vi "Teleop.vi"(10 "Match Info":T1={"Autonomous Elapsed Seconds"=0.0, "TeleOp Elapsed Seconds"=0.0, "Disabled Elapsed Seconds"=0.0, "Visited Autonomous"=FALSE, "Visited TeleOp"=FALSE, "Visited Disabled"=FALSE, "Autonomous Settings"={"Autonomous Style"=enum."Independent", "VI Refnum"=refnum}}, 11 "Call Context":T2) -> ()   [LabVIEW 2017]
doc: "This VI is called for each TeleOp packet received from the DS where the robot is not disabled. It is often used to read from the joysticks and update I/O or to update setpoints for timed control loops. It should complete and return within 20 milliseconds or it may miss DS packets."
uses:
  <vilib>/Rock Robotics/WPI/DriverStation/WPI_DriverStationDerivedRobotMode.ctl
  <vilib>/Rock Robotics/WPI/DriverStation/WPI_DriverStationMatch Info.ctl
  <vilib>/Rock Robotics/WPI/Solenoid/WPI_SolenoidValue.ctl
  <vilib>/Rock Robotics/WPI/Utilities/WPI_GetSetVariantRefNum.vi
  <vilib>/Rock Robotics/Network Tables/NT Write Boolean Array.vi
  <vilib>/Rock Robotics/Network Tables/NT Write Numeric Array.vi
  <vilib>/Rock Robotics/Network Tables/NT Read Boolean.vi
  <vilib>/Rock Robotics/Network Tables/NT Read Number.vi
  <vilib>/Rock Robotics/Network Tables/NT Write Number.vi
  <vilib>/Rock Robotics/WPI/Solenoid/WPI_SolenoidSetEnum.vi
panel:
  out "Sample Slider 0":dbl(slide) scale=0.0..5.0
  out "Sample Boolean 1":bool
  out "Sample Boolean 0":bool
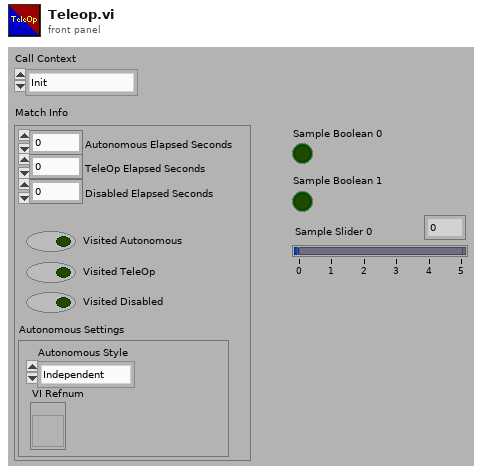
[diagram p1: front panel]
types:
  T1 = typedef "WPI_DriverStationMatch Info.ctl" = cluster{"Autonomous Elapsed Seconds":dbl, "TeleOp Elapsed Seconds":dbl, "Disabled Elapsed Seconds":dbl, "Visited Autonomous":bool, "Visited TeleOp":bool, "Visited Disabled":bool, "Autonomous Settings":cluster{"Autonomous Style":enum16{"Iterative", "Independent"}, "VI Refnum":refnum<vi>}}
  T2 = typedef "WPI_DriverStationDerivedRobotMode.ctl" = enum16{"Init", "Execute", "Stop"}
  T3 = typedef "WPI_SolenoidValue.ctl" = enum16{"Off", "On", "Forward", "Reverse"}
  T4 = typedef "WPI_JoystickDevRef.ctl" = cluster{"Device":T5}
  T5 = typedef "WPI_JoystickDeviceEnum.ctl" = enum16{"USB 0", "USB 1", "USB 2", "USB 3", "USB 4", "USB 5"}
  T6 = cluster{"Axes[0]":dbl, "Axes[1]":dbl, "Axes[2]":dbl, "Axes[3]":dbl, "Axes[4]":dbl, "Axes[5]":dbl, "Axes[6]":dbl, "Axes[7]":dbl, "Axes[8]":dbl}
  T7 = cluster{"Buttons[0]":bool, "Buttons[1]":bool, "Buttons[2]":bool, "Buttons[3]":bool, "Buttons[4]":bool, "Buttons[5]":bool, "Buttons[6]":bool, "Buttons[7]":bool, "Buttons[8]":bool}
  T8 = typedef "WPI_RobotDriveDevRef.ctl" = cluster{"DevStatus":errorcluster, "Motors[]":T9[], "Square Inputs":bool, "Max Output":dbl}
  T9 = typedef "WPI_MotorControlDeviceRef.ctl" = cluster{"DeviceStatus":errorcluster, "Type":T10, "PWM":cluster{"PWM Channel":T11, "DeadBand":T12}, "CAN":cluster{"Device Number":u8, "SetOutput VI Ref":variant, "GetOutput VI Ref":variant, "Enable VI Ref":variant, "Disable VI Ref":variant, "Data":variant}, "Invert":bool, "DIO PWM":cluster{"PWM \"Enable\" Channel":T11, "DIOChannel":T13, "PWM Rate":dbl}}
  T10 = typedef "WPI_MotorControlType.ctl" = enum16{"PWM", "CAN", "DIO PWM"}
  T11 = typedef "FPGA_DIOPWMChannel.ctl" = enum8{"PWM 0", "PWM 1", "PWM 2", "PWM 3", "PWM 4", "PWM 5", "PWM 6", "PWM 7", "PWM 8", "PWM 9", "PWM MXP 0", "PWM MXP 1", "PWM MXP 2", "PWM MXP 3", "PWM MXP 4", "PWM MXP 5", "PWM MXP 6", "PWM MXP 7", "PWM MXP 8", "PWM MXP 9", "Invalid"}
  T12 = typedef "WPI_PWMDeadband.ctl" = cluster{"Name":string, "maxPositivePwm":i32, "minPositivePwm":i32, "centerPwm":i32, "maxNegativePwm":i32, "minNegativePwm":i32, "angularRange":u16}
  T13 = typedef "FPGA_DIOChannel.ctl" = enum8{"DIO 0", "DIO 1", "DIO 2", "DIO 3", "DIO 4", "DIO 5", "DIO 6", "DIO 7", "DIO 8", "DIO 9", "DIO MXP 0", "DIO MXP 1", "DIO MXP 2", "DIO MXP 3", "DIO MXP 4", "DIO MXP 5", "DIO MXP 6", "DIO MXP 7", "DIO MXP 8", "DIO MXP 9", "DIO MXP 10", "DIO MXP 11", "DIO MXP 12", "DIO MXP 13", "DIO MXP 14", "DIO MXP 15", "SPI Port CS1", "SPI Port CS2", "SPI Port CS3", "SPI Port MISO", "SPI Port MOSI", "Invalid"}
  T14 = typedef "WPI_SolenoidDevRef.ctl" = cluster{"DevStatus":errorcluster, "Pneumatics Control Module":u8, "Forward Solenoid Channel":T15, "Reverse Solenoid Channel":T15}
  T15 = typedef "WPI_SolenoidChannel.ctl" = enum8{"Solenoid 0", "Solenoid 1", "Solenoid 2", "Solenoid 3", "Solenoid 4", "Solenoid 5", "Solenoid 6", "Solenoid 7", "Invalid"}
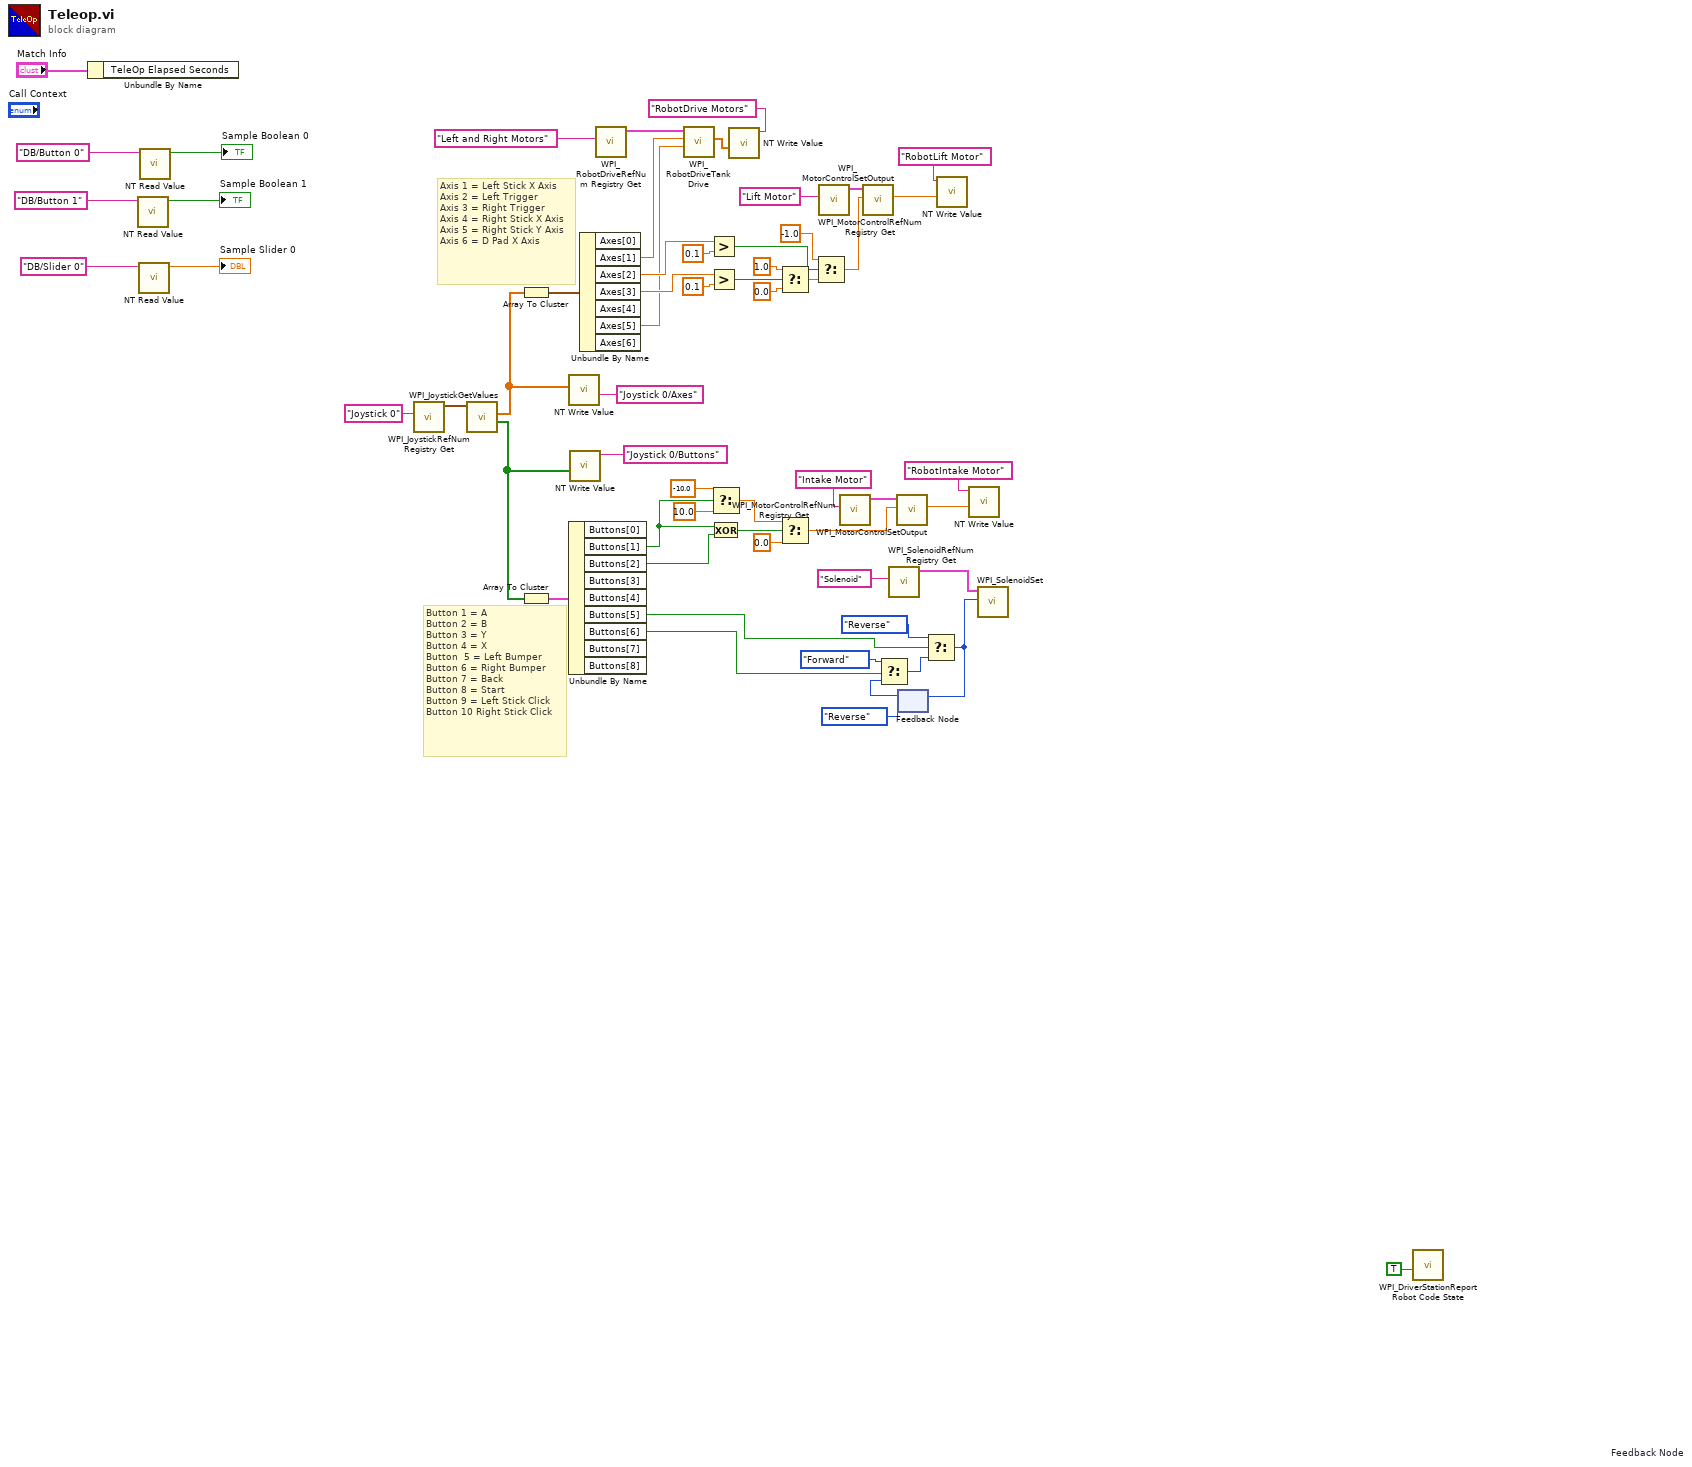
[diagram p0: block diagram]
diagram:
  # "Axis 1 = Left Stick X Axis\nAxis 2 = Left Trigger\nAxis 3 = Right Trigger\nAxis 4 = Right Stick X Axis\nAxis 5 = Right Stick Y Axis\nAxis 6 = D Pad X Axis"
  # "Button 1 = A\nButton 2 = B\nButton 3 = Y\nButton 4 = X\nButton  5 = Left Bumper\nButton 6 = Right Bumper\nButton 7 = Back\nButton 8 = Start\nButton 9 = Left Stick Click\nButton 10 Right Stick Click"
  n1 = Unbundle By Name("Match Info") -> ()  [unwired: 1 out]
  n2 = call-poly <vilib>:"NT Read Value.vi"("Name"="DB/Button 1" ("refnum name")) -> ("Boolean"=→"Sample Boolean 1":bool)  [unwired: 9 in, 1 out]
  n3 = call-poly <vilib>:"NT Read Value.vi"("Name"="DB/Slider 0" ("refnum name")) -> ("Numeric"=→"Sample Slider 0":dbl)  [unwired: 9 in, 1 out]
  n4 = call-poly <vilib>:"NT Read Value.vi"("Name"="DB/Button 0" ("refnum name")) -> ("Boolean"=→"Sample Boolean 0":bool)  [unwired: 9 in, 1 out]
  n5 = call <vilib>:"WPI_JoystickRefNum Registry Get.vi"("refnum name"="Joystick 0") -> ("JoystickDevRef"=w55:T4)  [unwired: 1 in, 9 out]
  n6 = call <vilib>:"WPI_JoystickGetValues.vi"("JoystickDevRef"=w55) -> ("Buttons"=w40:bool[], "Axes"=w43:dbl[])  [unwired: 6 in, 3 out]
  n7 = Array To Cluster(array=w43) -> (cluster=w42:T6)
  n8 = Array To Cluster(array=w40) -> (cluster=w39:T7)
  n9 = call-poly <vilib>:"NT Write Value.vi"("Numeric Array"=w43, "Name"="Joystick 0/Axes") -> ()  [unwired: 9 in, 1 out]
  n10 = Unbundle By Name(w39) -> ("Buttons[1]"=w3:bool, "Buttons[2]"=w4:bool, "Buttons[5]"=w2:bool, "Buttons[6]"=w1:bool)  [unwired: 5 out]
  n11 = call-poly <vilib>:"NT Write Value.vi"("Boolean Array"=w40, "Name"="Joystick 0/Buttons") -> ()  [unwired: 9 in, 1 out]
  n12 = Unbundle By Name(w42) -> ("Axes[1]"=w41:dbl, "Axes[2]"=w38:dbl, "Axes[3]"=w37:dbl, "Axes[5]"=w36:dbl)  [unwired: 3 out]
  n13 = call <vilib>:"WPI_RobotDriveRefNum Registry Get.vi"("refnum name"="Left and Right Motors") -> ("RobotDriveDevRef"=w57:T8)  [unwired: 1 in, 9 out]
  n14 = call <vilib>:"WPI_RobotDriveTankDrive.vi"("Right axis value"=w36, "Left axis value"=w41, "RobotDriveDevRef"=w57) -> ("Motor Values"=w45:dbl[])  [unwired: 6 in, 2 out]
  n15 = Greater?(x=w38, y=0.1) -> (0:w14:bool)
  n16 = Greater?(x=w37, y=0.1) -> (0:w16:bool)
  n17 = Select(t=-10.0, s=w3, f=10.0) -> (s? t:f=w33:dbl)
  n18 = Exclusive Or(1:w4, 2:w3) -> (0:w32:bool)
  n19 = call-poly <vilib>:"NT Write Value.vi"("Numeric Array"=w45, "Name"="RobotDrive Motors") -> ()  [unwired: 9 in, 1 out]
  n20 = Select(t=1.0, s=w16, f=0.0) -> (s? t:f=w21:dbl)
  n21 = Select(t=w33, s=w32, f=0.0) -> (s? t:f=w35:dbl)
  n22 = Select(t=-1.0, s=w14, f=w21) -> (s? t:f=w13:dbl)
  n23 = call <vilib>:"WPI_MotorControlRefNum Registry Get.vi"("refnum name"="Lift Motor") -> ("MotorControlDevRef"=w24:T9)  [unwired: 9 in, 1 out]
  n24 = call <vilib>:"WPI_MotorControlRefNum Registry Get.vi"("refnum name"="Intake Motor") -> ("MotorControlDevRef"=w30:T9)  [unwired: 9 in, 1 out]
  n25 = call <vilib>:"WPI_MotorControlSetOutput.vi"("Output"=w13, "MotorControlDevRef"=w24) -> ("Motor Output"=w23:dbl)  [unwired: 7 in, 2 out]
  n26 = call <vilib>:"WPI_SolenoidRefNum Registry Get.vi"("refnum name"="Solenoid") -> ("SolenoidDevRef"=w7:T14)  [unwired: 9 in, 1 out]
  n27 = call <vilib>:"WPI_MotorControlSetOutput.vi"("Output"=w35, "MotorControlDevRef"=w30) -> ("Motor Output"=w31:dbl)  [unwired: 7 in, 2 out]
  n28 = feedback #1 "Feedback Node"(WPI_SolenoidValue."Reverse" ("Value")) -> (w12:T3)
  n29 = Select(t=WPI_SolenoidValue."Forward" ("Value"), s=w1, f=w12) -> (s? t:f=w6:T3)
  n30 = Select(t=WPI_SolenoidValue."Reverse" ("Value"), s=w2, f=w6) -> (s? t:f=w10:T3)
  n31 = feedback-in #1(w10) -> ()
  n32 = call-poly <vilib>:"NT Write Value.vi"("Numeric"=w23, "Name"="RobotLift Motor") -> ()  [unwired: 9 in, 1 out]
  n33 = call-poly <vilib>:"NT Write Value.vi"("Numeric"=w31, "Name"="RobotIntake Motor") -> ()  [unwired: 9 in, 1 out]
  n34 = call-poly <vilib>:"WPI_SolenoidSet.vi"("Value"=w10, "SolenoidDevRef"=w7) -> ()  [unwired: 8 in, 2 out]
  n35 = call <vilib>:"WPI_DriverStationReport Robot Code State.vi"("TeleOp"=TRUE ("Autonomous")) -> ()  [unwired: 10 in, 1 out]
